vi "Hella CAN Gas.vi"(0 "Pressure Command (kPa)":u16, 11 "Error In":errorcluster) -> (4 "CAN Errors":dbl, 15 "Error Out":errorcluster)   [LabVIEW 2013]
uses:
  CAN Mode.ctl
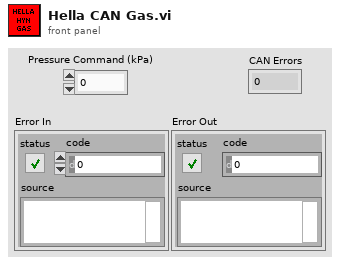
[diagram p1: front panel]
types:
  T1 = typedef "CAN Mode.ctl" = enum16{"Init", "Read", "Write", "Close"}
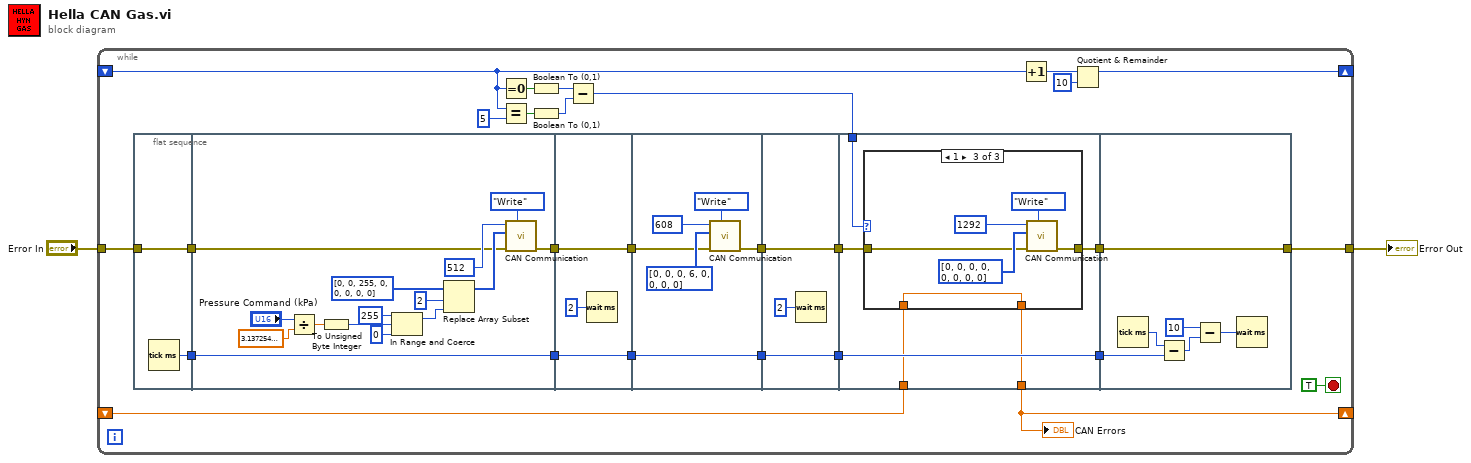
[diagram p0: block diagram]
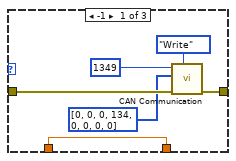
[diagram p2: hidden frame]
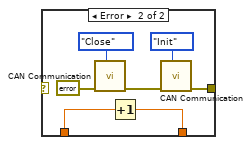
[diagram p4: hidden frame]
diagram:
  n1 = while {
    tunnel: "Error In" -> [w29]
    shift-right: [w16] -> _
    shift-left: _ -> [w15]
    tunnel: [w6] -> w1
    shift-right: [w3] -> _
    shift-left: _ -> [w4]
    stop <- TRUE stop-if-true
    n2 = flat-sequence {
      tunnel: w29 -> [w31]
      tunnel: [w31] -> w28
      tunnel: [w30] -> w8
      tunnel: w28 -> [w35]
      tunnel: [w34] -> w27
      tunnel: [w33] -> w9
      tunnel: w8 -> [w33]
      tunnel: w27 -> [w48]
      tunnel: [w48] -> w26
      tunnel: [w47] -> w10
      tunnel: w9 -> [w47]
      tunnel: w26 -> [w54]
      tunnel: [w53] -> w24
      tunnel: [w52] -> w11
      tunnel: w10 -> [w52]
      tunnel: [w57] -> w25
      tunnel: w24 -> [w57]
      tunnel: [w56] -> w12
      tunnel: w11 -> [w56]
      tunnel: w25 -> [w64]
      tunnel: w14 -> [w63]
      tunnel: [w62] -> w13
      tunnel: w12 -> [w62]
      tunnel: [w61] -> w5
      tunnel: w4 -> [w60]
      tunnel: [w59] -> w3
      tunnel: w13 -> [w95]
      tunnel: [w90] -> w6
      tunnel: w5 -> [w90]
      frame #0 {
        n3 = Tick Count (ms)() -> (millisecond timer value=w30:u32)
      }
      frame #1 {
        n4 = Divide(x="Pressure Command (kPa)", y=sgl 3.137255) -> (x/y=w39:sgl)
        n5 = To Unsigned Byte Integer(number=w39) -> (unsigned 8bit integer=w37:u8)
        n6 = In Range and Coerce(upper limit=u8 255, x=w37, lower limit=u8 0) -> (coerced(x)=w38:u8)  [unwired: 1 out]
        n7 = Replace Array Subset(array=u8[] [0, 0, 255, 0, 0, 0, 0, 0] ("Data Array (Hex) Bytes  0 -> 7"), new element=w38, index=2) -> (w45:u8[])
        n8 = call "CAN Communication.vi"("CAN Mode"=CAN_Mode."Write", "Error IN"=w35, "Message"=w45, "Arbitration ID"=u32 512) -> ("Error OUT"=w34:errorcluster)  [unwired: 6 in, 1 out]
      }
      frame #2 {
        n9 = Wait (ms)(milliseconds to wait=u32 2) -> ()  [unwired: 1 out]
      }
      frame #3 {
        n10 = call "CAN Communication.vi"("CAN Mode"=CAN_Mode."Write", "Error IN"=w54, "Message"=u8[] [0, 0, 0, 6, 0, 0, 0, 0] ("Data frame to 0x260"), "Arbitration ID"=u32 608 ("CAN Addres to Xmit\nSpeed CMD (Hex) 2")) -> ("Error OUT"=w53:errorcluster)  [unwired: 6 in, 1 out]
      }
      frame #4 {
        n11 = Wait (ms)(milliseconds to wait=u32 2) -> ()  [unwired: 1 out]
      }
      frame #5 {
        n12 = case shown="1" w63 {
          tunnel: w64 -> [w70 w74 w86]
          tunnel: [w68 w73 w85] -> w61
          tunnel: w60 -> [w65 w72 w84]
          tunnel: [w65 w71 w84] -> w59
          frame -1 {
            n13 = call "CAN Communication.vi"("CAN Mode"=CAN_Mode."Write", "Error IN"=w70, "Message"=u8[] [0, 0, 0, 134, 0, 0, 0, 0] ("Data frame to 0x545"), "Arbitration ID"=u32 1349) -> ("Error OUT"=w68:errorcluster)  [unwired: 6 in, 1 out]
          }
          frame Default {
            n14 = case shown="No Error" w74 {
              selector: w74 -> [w76 _]
              tunnel: [w76 w79] -> w73
              tunnel: w72 -> [w75 w78]
              tunnel: [w75 w77] -> w71
              frame No Error {
              }
              frame Error {
                n15 = call "CAN Communication.vi"("CAN Mode"=CAN_Mode."Close", "Error IN"=errorcluster {"status"=FALSE, "code"=0, "source"=""}) -> ("Error OUT"=w81:errorcluster)  [unwired: 8 in, 1 out]
                n16 = Increment(x=w78) -> (x+1=w77:dbl)
                n17 = call "CAN Communication.vi"("CAN Mode"=CAN_Mode."Init", "Error IN"=w81) -> ("Error OUT"=w79:errorcluster)  [unwired: 8 in, 1 out]
              }
            }
          }
          frame 1 {
            n18 = call "CAN Communication.vi"("CAN Mode"=CAN_Mode."Write", "Error IN"=w86, "Message"=u8[] [0, 0, 0, 0, 0, 0, 0, 0] ("Data frame to 0x50C"), "Arbitration ID"=u32 1292) -> ("Error OUT"=w85:errorcluster)  [unwired: 6 in, 1 out]
          }
        }
      }
      frame #6 {
        n19 = Tick Count (ms)() -> (millisecond timer value=w94:u32)
        n20 = Subtract(x=w94, y=w95) -> (x-y=w93:u32)
        n21 = Subtract(x=u32 10, y=w93) -> (x-y=w91:u32)
        n22 = Wait (ms)(milliseconds to wait=w91) -> ()  [unwired: 1 out]
      }
    }
    n23 = Equal To 0?(x=w15) -> (x = 0?=w20:bool)
    n24 = Equal?(x=w15, y=u32 5) -> (x = y?=w21:bool)
    n25 = Boolean To (0,1)(Boolean=w20) -> (0, 1=w22:i16)
    n26 = Boolean To (0,1)(Boolean=w21) -> (0, 1=w23:i16)
    n27 = Subtract(x=w22, y=w23) -> (x-y=w14:i16)
    n28 = Increment(x=w15) -> (x+1=w17:u32)
    n29 = Quotient & Remainder(x=w17, y=u32 10) -> (x-y*floor(x/y)=w16:u32)  [unwired: 1 out]
    "CAN Errors" <- w3
  }
  "Error Out" <- w1
